vi "AVERAGE OF N NUMBER.vi"() -> ()   [LabVIEW 2017]
panel:
  out "AVERAGE":dbl
  out "SUM":i32
  # "AVERAGE OF N NUMBER"
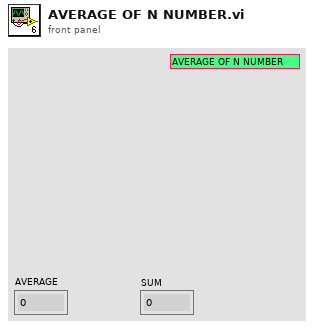
[diagram p1: front panel]
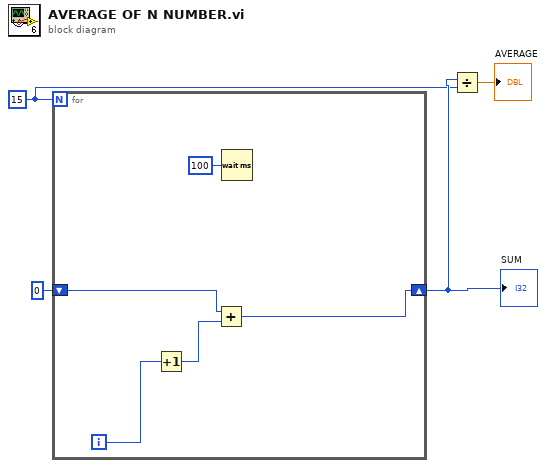
[diagram p0: block diagram]
diagram:
  w2 = 15
  n1 = for {
    N: w2 -> [_]
    shift-right: [w7] -> w3
    shift-left: 0 -> [w6]
    i -> [w9]
    n2 = Increment(x=w9) -> (x+1=w8:i32)
    n3 = Add(x=w6, y=w8) -> (x+y=w7:i32)
    n4 = Wait (ms)(milliseconds to wait=u32 100) -> ()  [unwired: 1 out]
  }
  "SUM" <- w3
  n5 = Divide(x=w3, y=w2) -> (x/y=→"AVERAGE":dbl)
